vi "Standard Type to Reflection.vi"(1 "Charact Standard":T2) -> (0 "Standard Type":T1 caption="Reflection" items=["Reflection 0", "Reflection 1", "Reflection 2", "Reflection 3", "Reflection 4", "Reflection 5", "Through 0", "Through 1"])   [LabVIEW 2023, in "NI Cal-5501 Cal Standard.lvlib" / "Cal Standard.lvclass"]
uses:
  Cal Standard.lvclass
  Cal Standard.lvclass/Cal Standard.ctl
  <instrlib>/niVCalModule/niVCalModule.llb/Standard Control.ctl
  Instruments/Cal Standard/Type Definitions/Standard Type.ctl
  Instruments/RFFixtureCharact.Instruments.lvlib
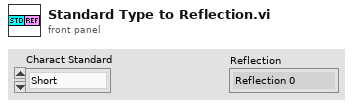
[diagram p1: front panel]
types:
  T1 = typedef "Standard Control.ctl" = i32
  T2 = typedef "RFFixtureCharact.Instruments.lvlib/Standard Type.ctl" = enum16{"Short", "Open", "Load", "PowerMeter", "None"}
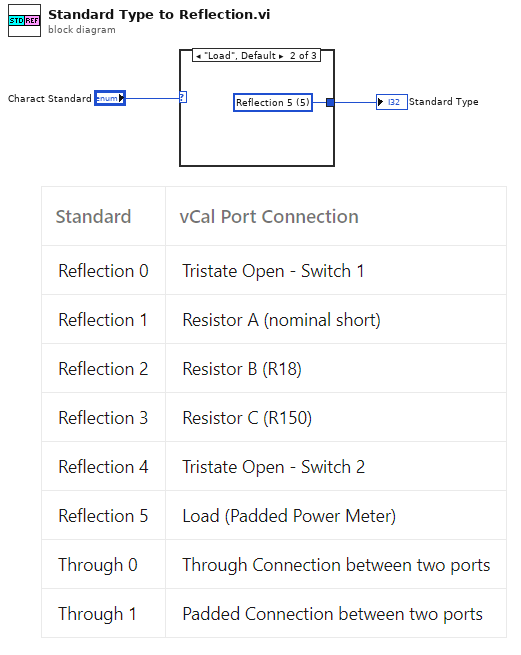
[diagram p0: block diagram]
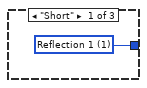
[diagram p2: hidden frame]
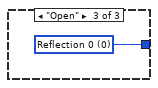
[diagram p3: hidden frame]
diagram:
  n1 = case shown="\"Load\", Default" "Charact Standard" {
    tunnel: [w3 w4 w5] -> w1
    frame "Short" {
      w3 = T1 1 items=["Reflection 0", "Reflection 1", "Reflection 2", "Reflection 3", "Reflection 4", "Reflection 5", "Through 0", "Through 1"] ("Standard")
    }
    frame "Load", Default {
      w4 = T1 5 items=["Reflection 0", "Reflection 1", "Reflection 2", "Reflection 3", "Reflection 4", "Reflection 5", "Through 0", "Through 1"] ("Standard")
    }
    frame "Open" {
      w5 = T1 0 items=["Reflection 0", "Reflection 1", "Reflection 2", "Reflection 3", "Reflection 4", "Reflection 5", "Through 0", "Through 1"] ("Standard")
    }
  }
  "Standard Type" <- w1
